vi "isma_speed.vi"() -> ()   [LabVIEW 2017]
uses:
  BERTTA.dll
panel:
  out "element":dbl format="%_6g"
  in  "port_mettler":i32=35
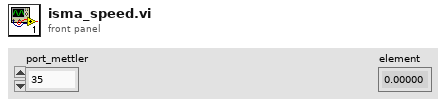
[diagram p1: front panel]
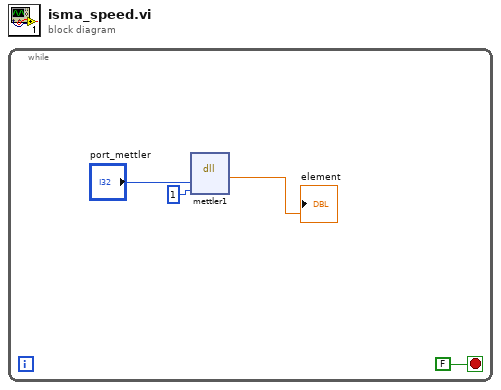
[diagram p0: block diagram]
diagram:
  n1 = while {
    stop <- FALSE stop-if-true
    n2 = dll-call lib="C:/Users/p3cn/OneDrive - Kemira Oyj/Documents/GitHub/Bertta/BERTTA/x64/Release/BERTTA.dll" fn="mettler1"("port_mettler"="port_mettler", "msg"=1) -> ("return type"=→"element":dbl)  [unwired: 5 in, 2 out]
  }
